vi "SwitchTest.vi"() -> ()   [LabVIEW 2012]
panel:
  out "Boolean":bool
  in  "switch":bool=TRUE
  # "momentary switch on pullup\npin -- normally high; pin push\npulls it low momentarily"
  # "when true motors run\nwhen false, stop"
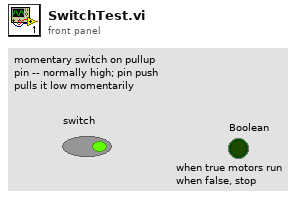
[diagram p1: front panel]
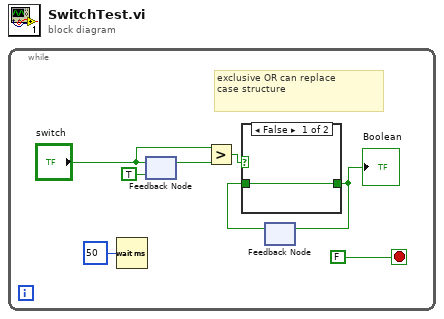
[diagram p0: block diagram]
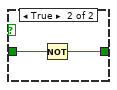
[diagram p2: hidden frame]
diagram:
  n1 = while {
    stop <- FALSE stop-if-true
    # "exclusive OR can replace\ncase structure"
    n2 = Wait (ms)(milliseconds to wait=u32 50) -> ()  [unwired: 1 out]
    n3 = feedback #1(TRUE ("switch")) -> (w8:bool)
    n4 = feedback-in #1("switch") -> ()
    n5 = Greater?(x="switch", y=w8) -> (0:w4:bool)
    n6 = feedback #2() -> (w3:bool)  [unwired: 1 in]
    n7 = case shown="False" w4 {
      tunnel: w3 -> [w9 w11]
      tunnel: [w9 w10] -> w2
      frame False {
      }
      frame True {
        n8 = Not(x=w11) -> (.not. x?=w10:bool)
      }
    }
    "Boolean" <- w2
    n9 = feedback-in #2(w2) -> ()
  }
